vi "scatch-vi.vi"() -> ()   [LabVIEW 2013]
panel:
  out "x+y 2":fxp<+,34,34> format="%b"
  out "x rotated left by y":u32 format="%b"
  out "x+y":fxp<+,33,33> format="%b"
  out "Boolean array":bool[](array[boolean])
  in  "F In":bool[](array[boolean])
  out "F Out":bool[](array[boolean])
  # "0011    000   1  000   1  0001     0000101101110100"
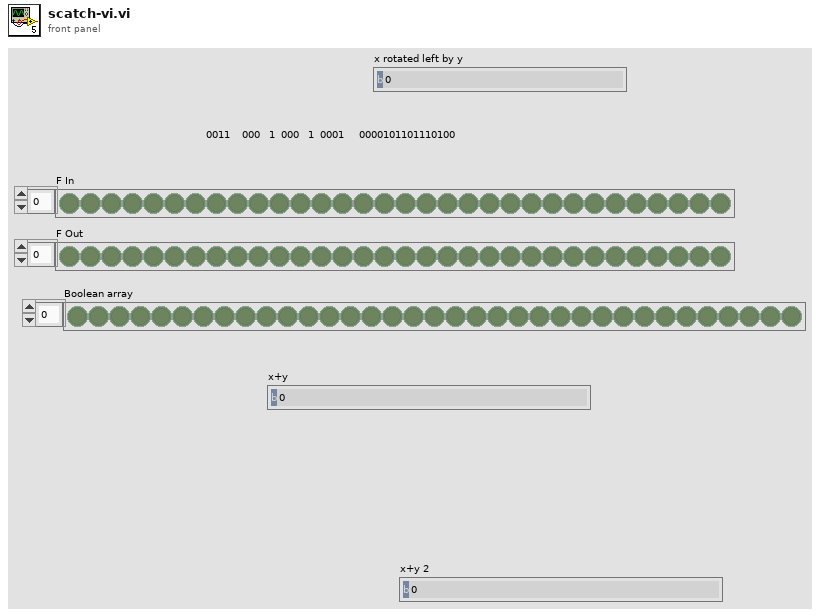
[diagram p1: front panel]
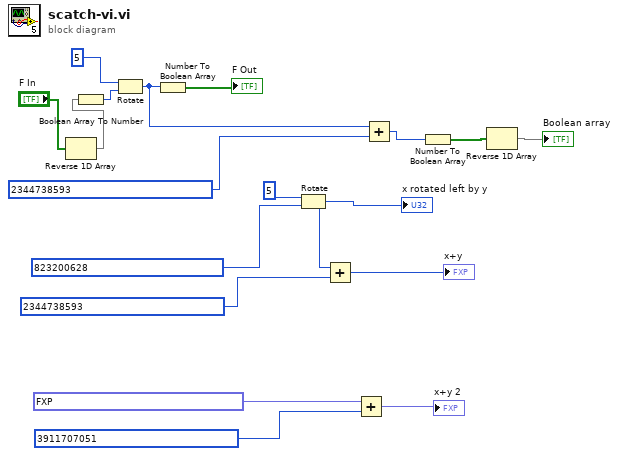
[diagram p0: block diagram]
diagram:
  n1 = Reverse 1D Array(array="F In") -> (reversed array=w12:bool[])
  n2 = Boolean Array To Number(Boolean array=w12) -> (number=w18:u32)
  n3 = Rotate(1:w18, 2:i16 5 ("y")) -> (0:w16:u32)
  n4 = Number To Boolean Array(number=w16) -> (Boolean array=→"F Out":bool[])
  n5 = Rotate(1:u32 823200628 ("y"), 2:i16 5 ("y")) -> (0:w5:u32)
  "x rotated left by y" <- w5
  n6 = Add(x=w5, y=u32 2344738593) -> (x+y=→"x+y":u32)
  n7 = Add(x=fxp<+,33,33> 7462906517.0 ("y"), y=u32 3911707051) -> (x+y=→"x+y 2":fxp<+,34,34>)
  n8 = Add(x=w16, y=u32 2344738593) -> (x+y=w14:u32)
  n9 = Number To Boolean Array(number=w14) -> (Boolean array=w11:bool[])
  n10 = Reverse 1D Array(array=w11) -> (reversed array=→"Boolean array":bool[])
